vi "2 digit number to 2 array.vi"(1 "Numeric":dbl format="%#_13g") -> (0 "transposed array":bool[][](array[boolean]))   [LabVIEW 2020]
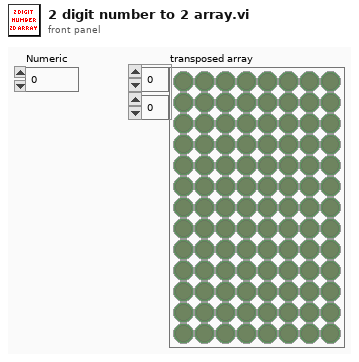
[diagram p1: front panel]
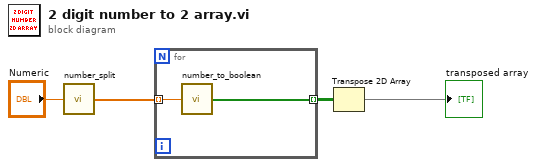
[diagram p0: block diagram]
diagram:
  n1 = call "number_split.vi"("Numeric"="Numeric") -> ("Split Numbers"=w2:dbl[])
  n2 = for {
    tunnel: w2 -> [w6] mode=indexing
    tunnel: [w5] -> w3 mode=indexing
    n3 = call "number_to_boolean.vi"("A in"=w6) -> ("A out"=w5:bool[])
  }
  n4 = Transpose 2D Array(2D array=w3) -> (transposed array=→"transposed array":bool[][])
